vi "Init Motor Config Obj by Label.vi"(8 "error in (no error)":errorcluster, 10 "Label":string, 11 "Motions Configuration in":refnum<class "Motions Configuration.lvclass">) -> (0 "error out":errorcluster, 1 "not found?":bool, 2 "Motor Configuration Obj":refnum<class "Motor Configuration.lvclass">, 3 "Motions Configuration out":refnum<class "Motions Configuration.lvclass">)   [LabVIEW 2016, in "Hardware.lvlib" / "Motions.lvlib" / "Motions Configuration.lvclass"]
uses:
  <userlib>/Common Components/Hardware/Abstract System/Motions/Motions Config/Motions Configuration.lvclass
  C:/Program Files (x86)/National Instruments/LabVIEW 2016/user.lib/Configuration Dialog Actor/Configuration.lvclass
  <userlib>/Common Components/Hardware/Motor/Motor Config/Motor Configuration.lvclass
  <userlib>/Common Components/Hardware/Abstract System/Motions/Motions Config/Motions Configuration.lvclass/Motions Configuration.ctl
  <userlib>/Configuration Dialog Actor/Configuration.lvclass/Configuration.ctl
  <userlib>/Common Components/Hardware/Abstract System/Motions/Motions/Motions.lvclass/Motions.ctl
  <userlib>/Common Components/Hardware/Abstract Hardware/Hardware.lvclass/Hardware.ctl
  <userlib>/Common Components/Hardware/Motor/Motor Config/Motor Configuration.lvclass/Motor Configuration.ctl
  <userlib>/Configuration Dialog Actor/Accessors/Write Change Display.vi
  <userlib>/Configuration Dialog Actor/Accessors/Write Sub Panel.vi
  <userlib>/Configuration Dialog Actor/Accessors/Write Title.vi
  <userlib>/Configuration Dialog Actor/Accessors/Write Categories.vi
  <userlib>/Common Components/Hardware/Abstract Hardware/Read Label.vi
  <userlib>/Common Components/Hardware/Abstract System/Motions/Motions Config/Read Motions Obj.vi
  <userlib>/Configuration Dialog Actor/Accessors/Read Change Display.vi
  <userlib>/Configuration Dialog Actor/Accessors/Read Sub Panel.vi
  <userlib>/Configuration Dialog Actor/Accessors/Read Title.vi
  <userlib>/Configuration Dialog Actor/Accessors/Read Categories.vi
  <userlib>/Common Components/Hardware/Motor/Motor/Motor.lvclass
  C:/Program Files (x86)/National Instruments/LabVIEW 2016/user.lib/Common Components/Hardware/Abstract Hardware/Hardware.lvclass
  <userlib>/Common Components/Hardware/Motor/Motor Config/Accessors/Write Motor Obj.vi
  <userlib>/Common Components/Hardware/Abstract System/Motions/Motions/Motions.lvclass
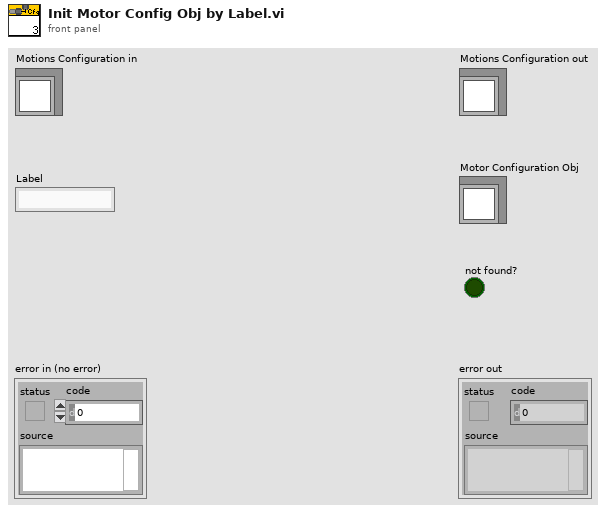
[diagram p1: front panel]
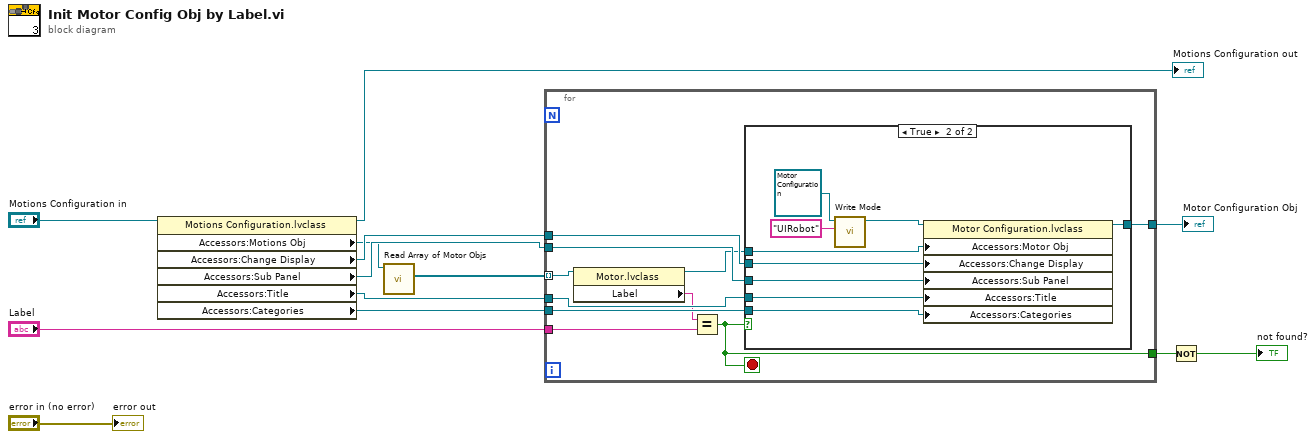
[diagram p0: block diagram]
diagram:
  n1 = property class="Motions Configuration.lvclass"(reference="Motions Configuration in") -> (reference out=→"Motions Configuration out":refnum<class "Motions Configuration.lvclass">, "Accessors:Motions Obj"=w8:refnum<class "Motions.lvclass">, "Accessors:Change Display"=w12:refnum<user-event>, "Accessors:Sub Panel"=w11:refnum<vi>, "Accessors:Title"=w10:refnum<vi>, "Accessors:Categories"=w9:refnum<vi>)  [unwired: 1 in, 1 out]
  n2 = call <userlib>:"Read Array of Motor Objs.vi"("Motions in"=w8) -> ("Array of Motor Objs"=w7:refnum<class "Motor.lvclass">[])  [unwired: 9 in, 1 out]
  n3 = for {
    tunnel: w12 -> [w23]
    tunnel: w11 -> [w22]
    tunnel: w10 -> [w21]
    tunnel: w9 -> [w20]
    tunnel: w7 -> [w19] mode=indexing
    tunnel: "Label" -> [w16]
    tunnel: [w15] -> w3
    tunnel: [w14] -> w2
    stop <- w14 stop-if-true
    n4 = property class="Motor.lvclass"(reference=w19) -> (reference out=w18:refnum<class "Motor.lvclass">, "Label"=w17:string)  [unwired: 1 in, 1 out]
    n5 = Equal?(x=w17, y=w16) -> (x = y?=w14:bool)
    n6 = case shown="True" w14 {
      tunnel: w23 -> [_ w32]
      tunnel: w22 -> [_ w31]
      tunnel: w21 -> [_ w30]
      tunnel: w20 -> [_ w29]
      tunnel: w18 -> [_ w24]
      tunnel: [_ w25] -> w15
      frame False {
      }
      frame True {
        n7 = call <userlib>:"Write Mode.vi"("Mode"="UIRobot", "Motor Configuration in"=refnum<class "Motor Configuration.lvclass"> refnum ("Motor Config Obj")) -> ("Motor Configuration out"=w27:refnum<class "Motor Configuration.lvclass">)  [unwired: 9 in]
        n8 = property class="Motor Configuration.lvclass"(reference=w27, "Accessors:Motor Obj"=w24, "Accessors:Change Display"=w32, "Accessors:Sub Panel"=w31, "Accessors:Title"=w30, "Accessors:Categories"=w29) -> (reference out=w25:refnum<class "Motor Configuration.lvclass">)  [unwired: 1 in, 1 out]
      }
    }
  }
  "Motor Configuration Obj" <- w3
  n9 = Not(x=w2) -> (.not. x?=→"not found?":bool)
  "error out" <- "error in (no error)"
